vi "Step a Motor.vi"(8 "error in (no error)":errorcluster, 9 "Dir":string(combo)="+", 10 "Index":i32, 11 "Motions in":refnum<class "Motions.lvclass">) -> (0 "error out":errorcluster, 3 "Motions out":refnum<class "Motions.lvclass">)   [LabVIEW 2016, in "Hardware.lvlib" / "Motions.lvlib" / "Motions.lvclass"]
uses:
  <userlib>/Common Components/Hardware/Abstract System/Motions/Motions/Motions.lvclass
  <userlib>/Common Components/Hardware/Abstract System/Motions/Motions/Motions.lvclass/Motions.ctl
  <userlib>/Common Components/Hardware/Motor/Motor/Motor.lvclass/Motor.ctl
  <userlib>/Common Components/Hardware/Motor/Motor/Accessor/Read max speed.vi
  <userlib>/Common Components/Hardware/Motor/Motor/Motor.lvclass
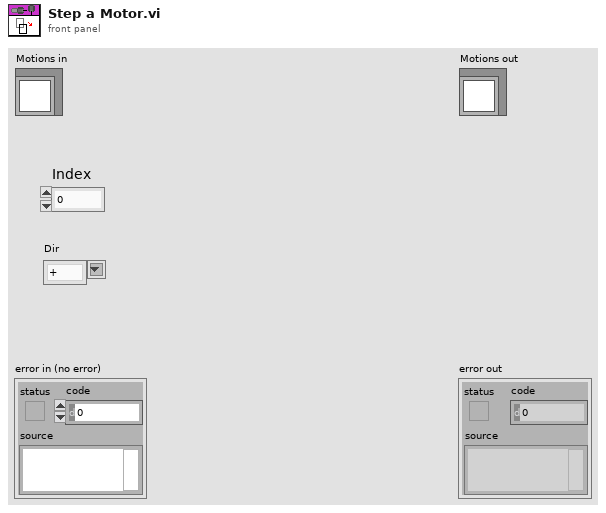
[diagram p1: front panel]
types:
  T1 = typedef "Hardware.lvlib/Motions.lvlib/Motions.lvclass/Motor States.ctl" = cluster{"Connected":bool, "Enabled":bool, "Moving Status":bool, "Soft Moving Status":bool, "Current Pos":dbl, "Target Pos":dbl, "Moving Dir (-1, 0, 1)":i32, "Error Status":bool, "Hard Limit+":bool, "Hard Limit-":bool, "Soft Limit+":bool, "Soft Limit-":bool, "History Dst Stack":refnum<queue>, "Motion Status":bool, "Motion TriggerAction Obj":refnum<class "TriggerAction Q.lvclass">}
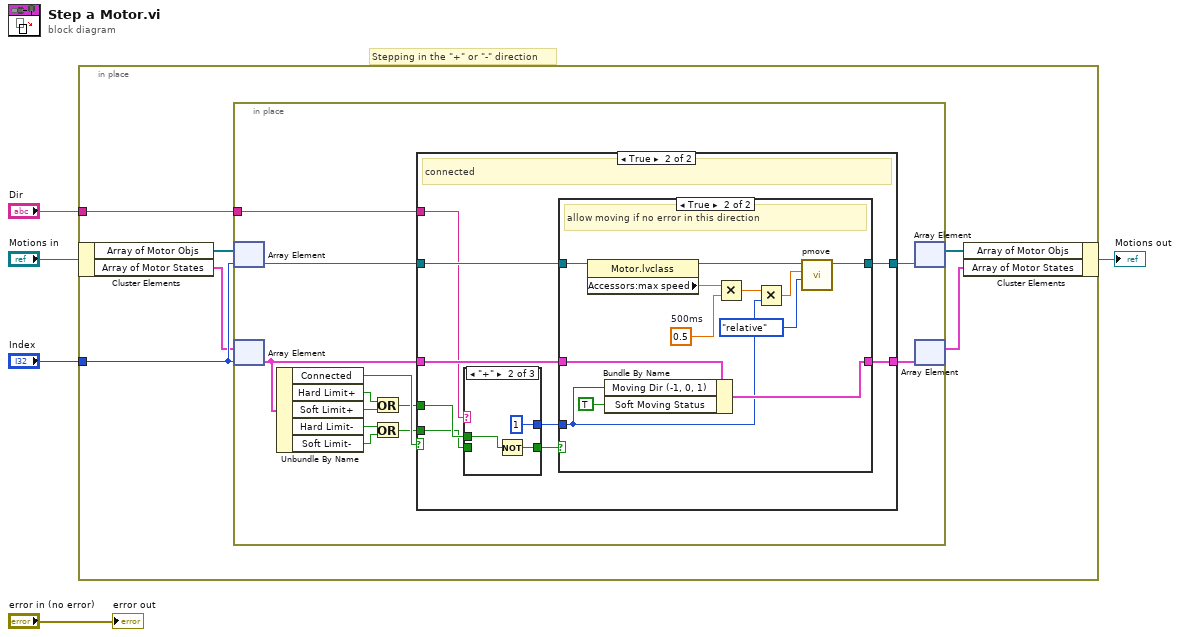
[diagram p0: block diagram]
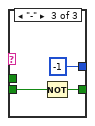
[diagram p4: hidden frame]
diagram:
  # "Stepping in the \"+\" or \"-\" direction"
  n1 = in-place {
    in-place-border: "Index" -> [w8]
    in-place-border: "Dir" -> [w9]
    n2 = in-place-cluster #1("Motions in") -> ("Array of Motor Objs"=w11:refnum<class "Motor.lvclass">[], "Array of Motor States"=w7:T1[])
    n3 = in-place {
      in-place-border: w9 -> [w22]
      n4 = in-place-array #2(w11, w8) -> (w23:refnum<class "Motor.lvclass">)
      n5 = in-place-array #3(w7, w8) -> (w21:T1)
      n6 = Unbundle By Name(w21) -> ("Connected"=w19:bool, "Hard Limit+"=w17:bool, "Soft Limit+"=w16:bool, "Hard Limit-"=w15:bool, "Soft Limit-"=w14:bool)
      n7 = Or(x=w17, y=w16) -> (x .or. y?=w13:bool)
      n8 = Or(x=w15, y=w14) -> (x .or. y?=w12:bool)
      n9 = case shown="True" w19 {
        tunnel: w23 -> [w24 w32]
        tunnel: w22 -> [_ w27]
        tunnel: w21 -> [w25 w34]
        tunnel: [w25 w33] -> w20
        tunnel: [w24 w31] -> w18
        tunnel: w13 -> [_ w29]
        tunnel: w12 -> [_ w28]
        frame False {
        }
        frame True {
          # "connected"
          n10 = case shown="\"+\"" w27 {
            tunnel: [_ w36 w39] -> w30
            tunnel: w29 -> [_ w37 _]
            tunnel: w28 -> [_ _ w40]
            tunnel: [_ 1 -1] -> w26
            frame Default {
            }
            frame "+" {
              n11 = Not(x=w37) -> (.not. x?=w36:bool)
            }
            frame "-" {
              n12 = Not(x=w40) -> (.not. x?=w39:bool)
            }
          }
          n13 = case shown="True" w30 {
            tunnel: w26 -> [_ w43]
            tunnel: w34 -> [w41 w54]
            tunnel: [w41 w53] -> w33
            tunnel: w32 -> [w42 w50]
            tunnel: [w42 w52] -> w31
            frame False {
            }
            frame True {
              w46 = 0.5  # 500ms
              # "allow moving if no error in this direction"
              n14 = property class="Motor.lvclass"(reference=w50) -> (reference out=w49:refnum<class "Motor.lvclass">, "Accessors:max speed"=w47:dbl)  [unwired: 1 in, 1 out]
              n15 = Bundle By Name(cluster=w54, "Moving Dir (-1, 0, 1)"=w43, "Soft Moving Status"=TRUE) -> (w53:T1)
              n16 = Multiply(x=w47, y=w46) -> (x*y=w45:dbl)
              n17 = Multiply(x=w45, y=w43) -> (x*y=w44:dbl)
              n18 = call <userlib>:"pmove.vi"("mode (0: rel; 1: abs)"=enum16{"relative", "absolute"}."relative", "distance in display unit"=w44, "Motor in"=w49) -> ("Motor out"=w52:refnum<class "Motor.lvclass">)  [unwired: 7 in, 1 out]
            }
          }
        }
      }
      n19 = in-place-array #2(w18) -> (w10:refnum<class "Motor.lvclass">[])  [unwired: 1 out]
      n20 = in-place-array #3(w20) -> (w6:T1[])  [unwired: 1 out]
    }
    n21 = in-place-cluster #1("Array of Motor Objs"=w10, "Array of Motor States"=w6) -> (→"Motions out":refnum<class "Motions.lvclass">)
  }
  "error out" <- "error in (no error)"
